vi "Handle Message.vi"(7 "priority":T1, 8 "error in (no error)":errorcluster, 10 "Message":refnum<class "Message.lvclass">, 11 "Pub Sub Retaining Message Channel in":refnum<class "Pub Sub Retaining Message Channel.lvclass">) -> (0 "error out":errorcluster)   [LabVIEW 2020, in "Actor Pub Sub Channels.lvlib" / "Pub Sub Retaining Message Channel.lvclass"]
uses:
  Pub Sub Retaining Message Channel.lvclass
  <vilib>/ActorFramework/Message Dequeuer/Dequeue Priority.ctl
  <vilib>/ActorFramework/Message/Message.lvclass
  Pub Sub Retaining Message Channel.lvclass/Pub Sub Retaining Message Channel.ctl
  Pub Sub Status Message/Pub Sub Status Message.lvclass
  Pub Sub Message Channel/Pub Sub Message Channel.lvclass
  <vilib>/ActorFramework/Message Dequeuer/Message Dequeuer.lvclass
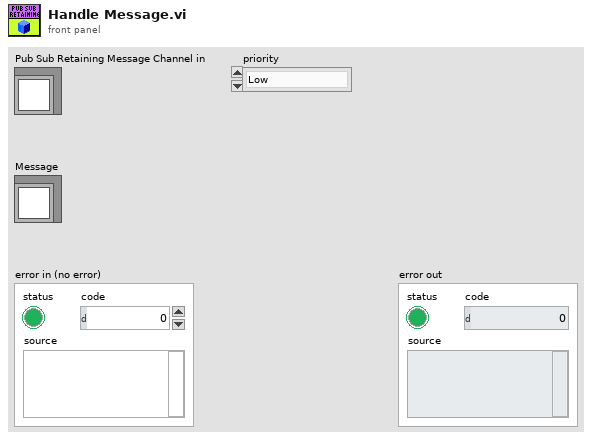
[diagram p1: front panel]
types:
  T1 = typedef "Actor Framework.lvlib/Message Dequeuer.lvclass/Dequeue Priority.ctl" = enum16{"Low", "Normal", "High", "Critical"}
  T2 = cluster{"Actor Framework:Message":refnum<class "Message.lvclass">}
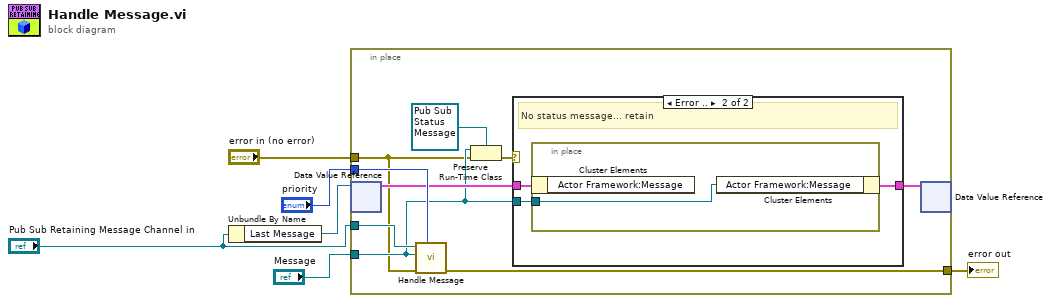
[diagram p0: block diagram]
diagram:
  n1 = Unbundle By Name("Pub Sub Retaining Message Channel in") -> ("Last Message"=w1:refnum<data-value>)
  n2 = in-place {
    in-place-border: [w15] -> w6
    in-place-border: "priority" -> [w14]
    in-place-border: "error in (no error)" -> [w7]
    in-place-border: "Message" -> [w10]
    in-place-border: "Pub Sub Retaining Message Channel in" -> [w13]
    n3 = in-place-dvr #1(w1) -> (w12:T2)  [unwired: 1 out]
    n4 = call-parent "Handle Message.vi"("priority"=w14, "error in (no error)"=w7, "Message"=w10, "Pub Sub Message Channel in"=w13) -> ("error out"=w15:errorcluster)  [unwired: 7 in]
    n5 = Preserve Run-Time Class(object in=w10, error in=w7, 2:refnum<class "Pub Sub Status Message.lvclass"> refnum ("Actor Pub Sub Channels.lvlib:Pub Sub Status Message.lvclass")) -> (error out=w8:errorcluster)  [unwired: 1 out]
    n6 = case shown="Error .." w8 {
      tunnel: w12 -> [w16 w19]
      tunnel: [w16 w18] -> w11
      tunnel: w10 -> [_ w17]
      frame No Error {
        # "just a status message. ignore"
      }
      frame Error {
        # "No status message... retain"
        n7 = in-place {
          in-place-border: w17 -> [w20]
          n8 = in-place-cluster #2(w19) -> ()  [unwired: 1 out]
          n9 = in-place-cluster #2("Actor Framework:Message"=w20) -> (w18:T2)
        }
      }
    }
    n10 = in-place-dvr #1(w11) -> ()  [unwired: 2 out]
  }
  "error out" <- w6
